vi "Init.vi"(8 "error in (no error)":errorcluster, 10 "Price":dbl, 11 "Bed in":refnum<class "Bed.lvclass">) -> (0 "error out":errorcluster, 3 "Bed out":refnum<class "Bed.lvclass">)   [LabVIEW 2019, in "Bed.lvclass"]
uses:
  Bed.lvclass
  Furniture.lvclass
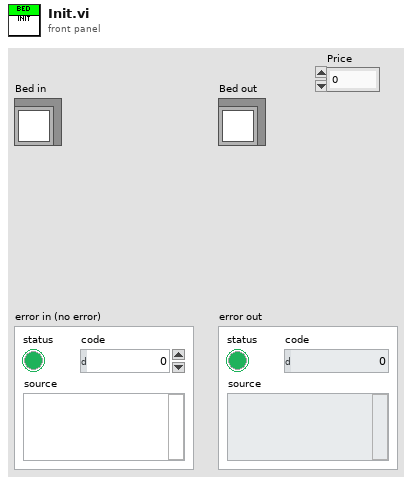
[diagram p1: front panel]
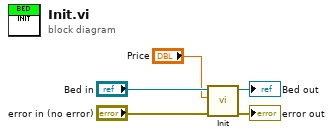
[diagram p0: block diagram]
diagram:
  n1 = call-parent "Init.vi"("error in (no error)"="error in (no error)", "Price"="Price", "Furniture in"="Bed in") -> ("error out"=→"error out":errorcluster, "Furniture out"=→"Bed out":refnum<class "Bed.lvclass">)  [unwired: 7 in]
